vi "CreateNewSheet.vi"(8 "error in (no error)":errorcluster, 10 "SheetName":string, 11 "Refnum Cluster In":T1) -> (0 "error out":errorcluster, 3 "Refnum Cluster Out":T2)   [LabVIEW 2015]
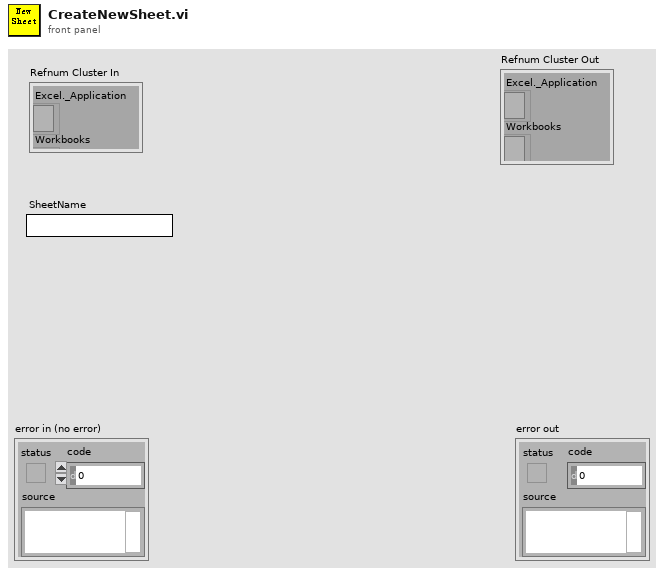
[diagram p1: front panel]
types:
  T1 = cluster{"Excel._Application":refnum<k7>, "Workbooks":refnum<k7>, "Open":refnum<k7>}
  T2 = cluster{"Excel._Application":refnum<k7>, "Workbooks":refnum<k7>, "Open":refnum<k7>, "Worksheets":refnum<k7>, "Excel._Worksheet":refnum<k7>}
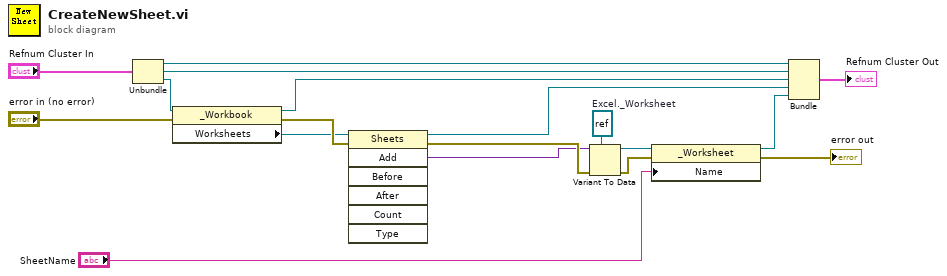
[diagram p0: block diagram]
diagram:
  w15 = refnum<k7> refnum  # Excel._Worksheet
  n1 = Unbundle("Refnum Cluster In") -> ("Excel._Application"=w12:refnum<k7>, "Workbooks"=w13:refnum<k7>, "Open"=w11:refnum<k7>)
  n2 = property class="_Workbook"(reference=w11, error in="error in (no error)") -> (reference out=w18:refnum<k7>, error out=w16:errorcluster, "Worksheets"=w7:refnum<k7>)
  n3 = invoke class="Sheets" method="Add"(reference=w7, error in=w16) -> (reference out=w6:refnum<k7>, error out=w17:errorcluster, "Add"=w14:variant)  [unwired: 5 in, 4 out]
  n4 = Variant To Data(error in=w17, type=w15, Variant=w14) -> (data=w5:refnum<k7>, error out=w3:errorcluster)
  n5 = property class="_Worksheet"(reference=w5, error in=w3, "Name"="SheetName") -> (reference out=w2:refnum<k7>, error out=→"error out":errorcluster)
  n6 = Bundle("Excel._Application"=w12, "Workbooks"=w13, "Open"=w18, "Worksheets"=w6, "Excel._Worksheet"=w2) -> (→"Refnum Cluster Out":T2)  [unwired: 1 in]
